vi "PID motor STEP.vi"() -> ()   [LabVIEW 2012]
panel:
  out "step":dbl
  in  "step":dbl(slide)=3.1518595041322315 scale=2.0..3.25
  out "error":dbl(slide) scale=-5.0..5.0
  out "error":dbl
  out "Td 3":dbl=0.3305785123966942
  out "kp 3":dbl=0.24793388429752067
  out "Td 2":dbl=0.43388429752066116
  in  "Ti":dbl(slide)=0.4132231404958678 scale=0.0..5.0
  in  "Td":dbl(slide)=0.3305785123966942 scale=0.0..5.0
  in  "Kp":dbl(slide)=0.3925619834710744 scale=0.0..5.0
  out "Respuesta del sistema":dynamicdata(graph)
  in  "T":dbl=0.019
  in  "OFF":bool
  # "VARIABLES DEL CONTROL PID"
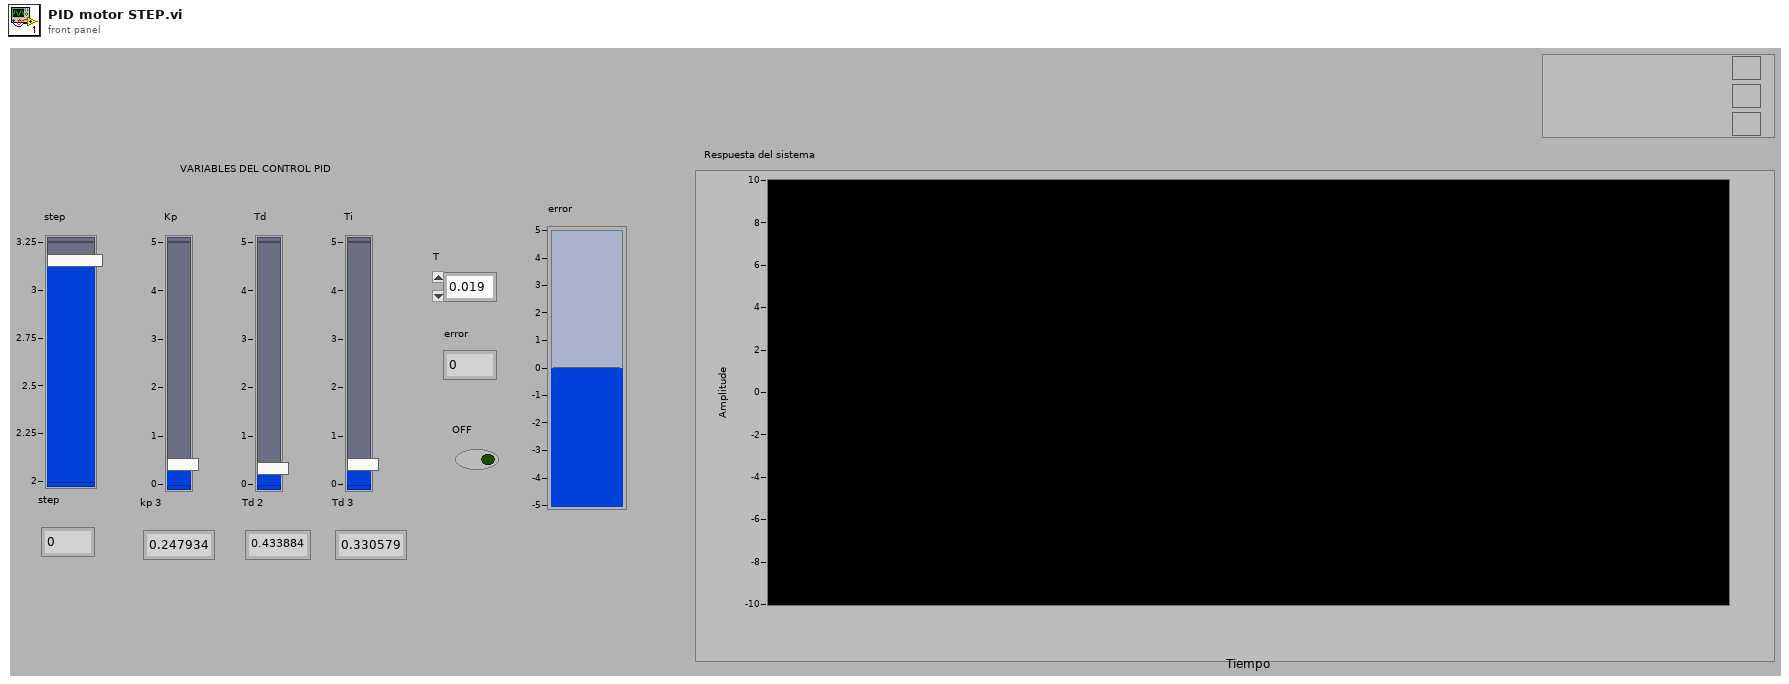
[diagram p1: front panel]
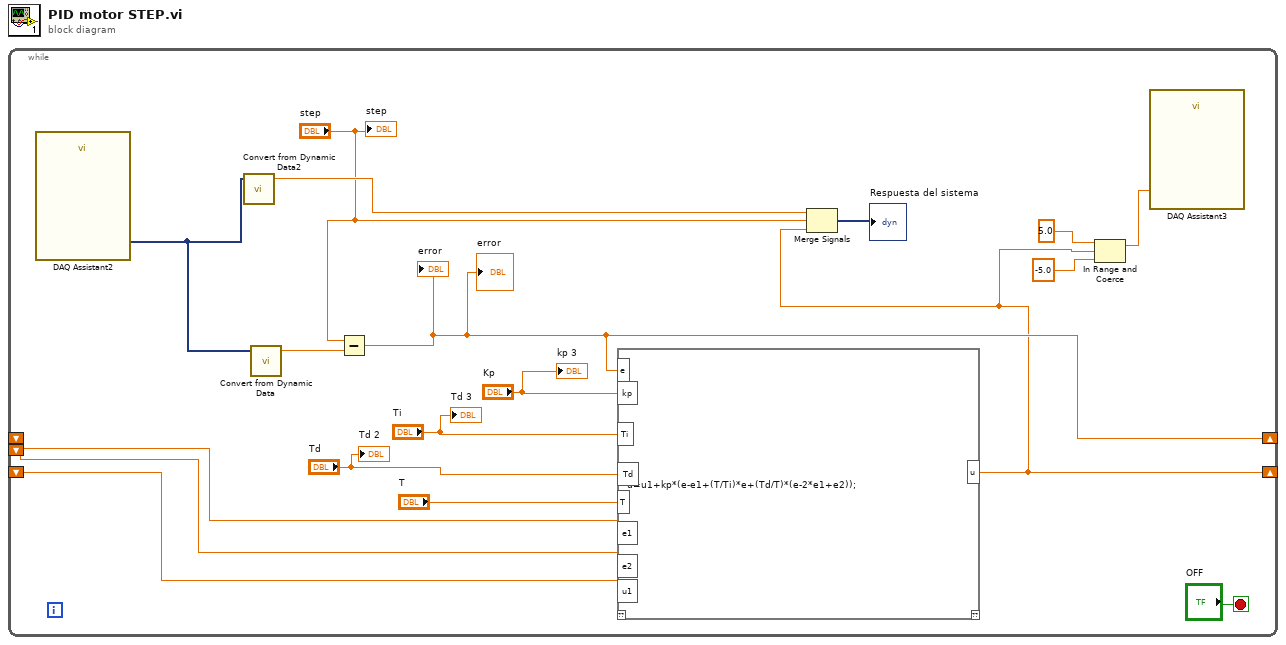
[diagram p0: block diagram]
diagram:
  n1 = while {
    shift-right: [w1] -> _
    shift-left: _ -> [w18]
    shift-right: [w5] -> _
    shift-left: _ -> [w17]
    shift-left: _ -> [w16]
    stop <- "OFF" stop-if-true
    n2 = call "DAQ Assistant2"() -> ("data"=w4:dynamicdata)  [unwired: 17 in, 2 out]
    n3 = call "Convert from Dynamic Data2"("Dynamic Data Type"=w4) -> ("Scalar"=w3:dbl)  [unwired: 3 in]
    n4 = call "Convert from Dynamic Data"("Dynamic Data Type"=w4) -> ("Scalar"=w13:dbl)  [unwired: 3 in]
    n5 = Subtract(x="step", y=w13) -> (x-y=w5:dbl)
    "error" <- w5
    "error" <- w5
    n6 = script code="u=u1+kp*(e-e1+(T/Ti)*e+(Td/T)*(e-2*e1+e2));"("kp"="Kp", "Ti"="Ti", "Td"="Td", "T"="T", "e2"=w16, "e"=w5, "u1"=w18, "e1"=w17) -> ("u"=w1:dbl)  [unwired: 1 in, 1 out]
    n7 = Merge Signals(w3, "step", w1) -> (→"Respuesta del sistema":dynamicdata)
    n8 = In Range and Coerce(upper limit=5.0, x=w1, lower limit=-5.0) -> (coerced(x)=w9:dbl)  [unwired: 1 out]
    n9 = call "DAQ Assistant3"("data"=w9) -> ()  [unwired: 17 in, 2 out]
    "Td 2" <- "Td"
    "kp 3" <- "Kp"
    "Td 3" <- "Ti"
    "step" <- "step"
  }
